vi "SCLN_ServerReadWriteMessage5.vi"(2 "error in (no error)":errorcluster, 3 "Client Number":i32 min=0 max=50, 4 "Server Number":i32, 5 "TCP ID In":refnum<k5>) -> (0 "error out":errorcluster, 1 "TCP ID Out":refnum<k5>)   [LabVIEW 2015]
doc: "Read a message sent from a TCP/IP\nclient to a server. The VI receives the\nmessages and pass the data to\nthe user by means of a queue. The VI\nthen waits on another queue for the\nuser response, that gets routed to\nthe original client.\nThe VI is exited either because of\nerror condition or shutdown\nnotification.\n\nThe message consists of 4 bytes\nwith the lenght of the message and\nthen the data."
uses:
  SCLN_RW_Select.ctl
panel:
  out "Error mess":string
  out "Data In":string
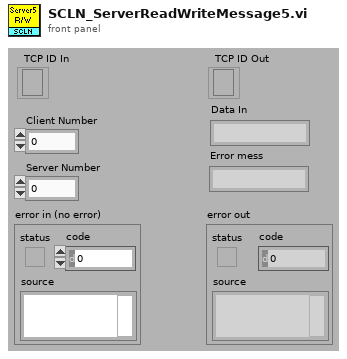
[diagram p1: front panel]
types:
  T1 = typedef "SCLN_RW_Select.ctl" = enum16{"Read", "Write"}
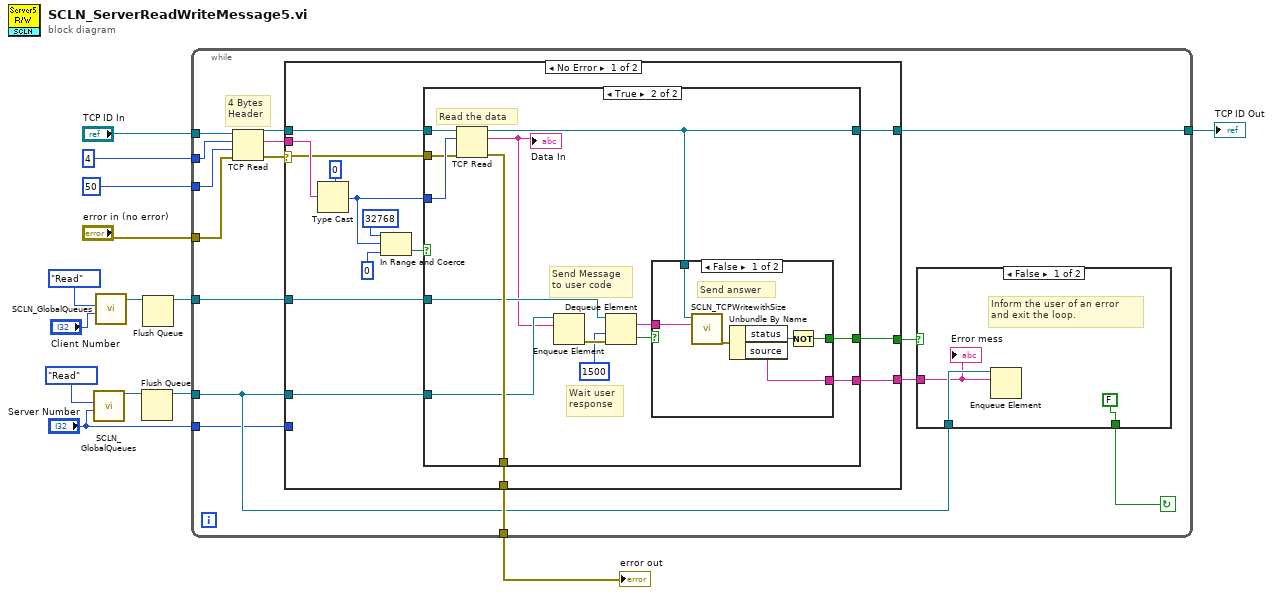
[diagram p0: block diagram]
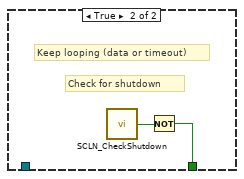
[diagram p2: hidden frame]
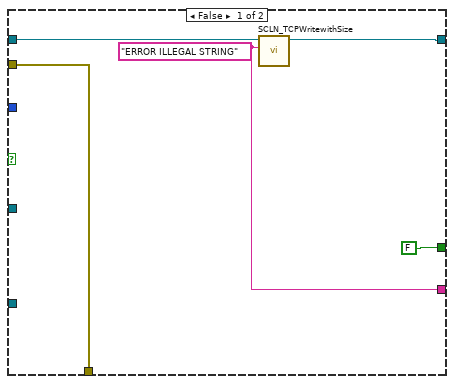
[diagram p3: hidden frame]
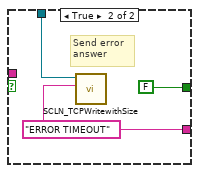
[diagram p4: hidden frame]
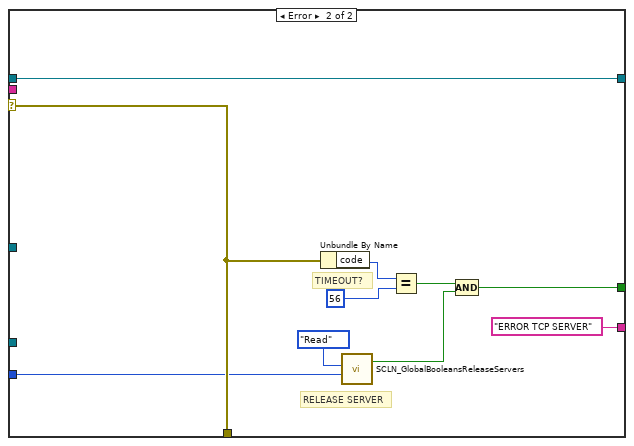
[diagram p5: hidden frame]
diagram:
  n1 = call "SCLN_GlobalQueues.vi"("Element"="Server Number", "Operation"=SCLN_RW_Select."Read" ("GBL_RW")) -> ("Read QueueID"=w3:refnum<queue>)  [unwired: 6 in, 1 out]
  n2 = call "SCLN_GlobalQueues.vi"("Element"="Client Number", "Operation"=SCLN_RW_Select."Read" ("GBL_RW")) -> ("Read QueueID"=w5:refnum<queue>)  [unwired: 6 in, 1 out]
  n3 = Flush Queue(queue=w3) -> (queue out=w2:refnum<queue>)  [unwired: 1 in, 2 out]
  n4 = Flush Queue(queue=w5) -> (queue out=w4:refnum<queue>)  [unwired: 1 in, 2 out]
  n5 = while {
    tunnel: "TCP ID In" -> [w29]
    tunnel: 4 ("bytes to read") -> [w28]
    tunnel: 50 ("timeout ms (25000)") -> [w27]
    tunnel: "error in (no error)" -> [w26]
    tunnel: [w20] -> w10
    tunnel: [w19] -> w9
    tunnel: w4 -> [w18]
    tunnel: w2 -> [w17]
    tunnel: "Server Number" -> [w15]
    stop <- w21 continue-if-true
    # "4 Bytes\nHeader"
    n6 = TCP Read(connection ID=w29, bytes to read=w28, error in (no error)=w26, 9:w27) -> (connection ID out=w25:refnum<k5>, data out=w24:string, error out=w16:errorcluster)  [unwired: 1 in]
    n7 = case shown="No Error" w16 {
      selector: w16 -> [w38 w79]
      tunnel: w25 -> [w48 w86]
      tunnel: w24 -> [w46 _]
      tunnel: [w41 w80] -> w23
      tunnel: [w45 w86] -> w20
      tunnel: [w37 "ERROR TCP SERVER"] -> w22
      tunnel: [w44 w79] -> w19
      tunnel: w18 -> [w43 _]
      tunnel: w17 -> [w42 _]
      tunnel: w15 -> [_ w78]
      frame No Error {
        n8 = Type Cast(type=0, x=w46) -> (*(type *) &x=w39:i32)
        n9 = In Range and Coerce(upper limit=32768, x=w39, lower limit=0) -> (In Range?=w40:bool)  [unwired: 1 out]
        n10 = case shown="True" w40 {
          tunnel: w48 -> [w53 w67]
          tunnel: [w52 w66] -> w45
          tunnel: [w51 w65] -> w44
          tunnel: w43 -> [_ w56]
          tunnel: w42 -> [_ w63]
          tunnel: [FALSE w62] -> w41
          tunnel: w39 -> [_ w61]
          tunnel: w38 -> [w51 w57]
          tunnel: [w50 w54] -> w37
          frame False {
            w50 = "ERROR ILLEGAL STRING"
            n11 = call "SCLN_TCPWritewithSize.vi"("data in"=w50, "connection ID"=w53) -> ("connection ID out"=w52:refnum<k5>)  [unwired: 7 in, 2 out]
          }
          frame True {
            # "Wait user\nresponse"
            # "Send Message\nto user code"
            # "Read the data"
            n12 = TCP Read(connection ID=w67, bytes to read=w61, error in (no error)=w57) -> (connection ID out=w66:refnum<k5>, data out=w55:string, error out=w65:errorcluster)  [unwired: 2 in]
            "Data In" <- w55
            n13 = Enqueue Element(queue=w63, element=w55) -> (error out=w64:errorcluster)  [unwired: 2 in, 2 out]
            n14 = Dequeue Element(queue=w56, timeout in ms (-1)=1500, error in (no error)=w64) -> (element=w59:string, timed out?=w58:bool)  [unwired: 2 out]
            n15 = case shown="False" w58 {
              tunnel: w66 -> [w73 w75]
              tunnel: w59 -> [w72 _]
              tunnel: [w69 FALSE] -> w62
              tunnel: [w68 w74] -> w54
              frame False {
                # "Send answer"
                n16 = call "SCLN_TCPWritewithSize.vi"("data in"=w72, "connection ID"=w73) -> ("error out"=w71:errorcluster)  [unwired: 7 in, 2 out]
                n17 = Unbundle By Name(w71) -> ("status"=w70:bool, "source"=w68:string)
                n18 = Not(x=w70) -> (.not. x?=w69:bool)
              }
              frame True {
                w74 = "ERROR TIMEOUT"
                # "Send error\nanswer"
                n19 = call "SCLN_TCPWritewithSize.vi"("data in"=w74, "connection ID"=w75) -> ()  [unwired: 7 in, 3 out]
              }
            }
          }
        }
      }
      frame Error {
        # "RELEASE SERVER"
        # "TIMEOUT?"
        n20 = Unbundle By Name(w79) -> ("code"=w84:i32)
        n21 = call "SCLN_GlobalBooleansReleaseServers.vi"("Element"=w78, "Operation"=SCLN_RW_Select."Read" ("GBL_RW")) -> ("Read Value"=w77:bool)  [unwired: 2 in, 1 out]
        n22 = Equal?(x=w84, y=56) -> (x = y?=w81:bool)
        n23 = Compound Arithmetic op=AND(w81, w77) -> (w80:bool)
      }
    }
    n24 = case shown="False" w23 {
      tunnel: [FALSE w33] -> w21
      tunnel: w22 -> [w30 _]
      tunnel: w17 -> [w31 _]
      frame False {
        # "Inform the user of an error\nand exit the loop."
        n25 = Enqueue Element(queue=w31, element=w30) -> ()  [unwired: 2 in, 3 out]
        "Error mess" <- w30
      }
      frame True {
        # "Keep looping (data or timeout)"
        # "Check for shutdown"
        n26 = call "SCLN_CheckShutdown.vi"() -> ("Shutdown"=w34:bool)
        n27 = Not(x=w34) -> (.not. x?=w33:bool)
      }
    }
  }
  "TCP ID Out" <- w10
  "error out" <- w9
